vi "config_LS218_CRYO_FDS.vi"(8 "entrée d'erreur":errorcluster, 11 "Port_COM":refnum<visa-resource-name>) -> (0 "sortie d'erreur":errorcluster)   [LabVIEW 2016]
panel:
  out "conf_OK":bool
  out "conf_check":bool[](array[boolean])
  in  "VERIFIER CONFIG":bool
  out "LECTURE BUFFER":bool
  out "LOAD":string
  in  "Type sondes 5-8":u16(ring) items=["Diode 2.5V", "Diode 7.5V", "Pt < 250 Ohm", "Pt < 500 Ohm", "Pt < 5 KOhm", "Cernox"]
  in  "Type sondes 1-4":u16(ring) items=["Diode 2.5V", "Diode 7.5V", "Pt < 250 Ohm", "Pt < 500 Ohm", "Pt < 5 KOhm", "Cernox"]
  in  "Voies de mesures":T1(array[cluster]) {"Input_type" items=["aucune", "DT-470 (diode)", "DT-500 (diode)", "CTI (diode)", "DT- 670 (diode)", "Cernox", "Pt100", "Pt1000"]}
  out "nombre renvoyé":u32
  in  "SEND":bool
  out "RÉPONSE":string
  in  "COMMANDE":string
  in  "Celsius":bool
  in  "PÉRIODE ACQUISITION (sec)":i8(slide)=1 min=1 max=60 step=1 scale=1.0..60.0
  in  "NOM MANIP":string="Cryo FDS"
  in  "QUITTER":bool
  in  "DOSSIER":path=path "C:/Fete de la science"
  in  "Acquisition":bool
  # "ACQUISITION LAKESHORE 218 : CONFIGURATION"
  # "PARAMÈTRES D'ACQUISITION"
  # "J. HANSOTTE - IAS\nStation d'Étalonnage"
  # "ÉTAT LIAISON RS232"
  # "D'ENREGISTREMENT DES MESURES"
  # "UNITÉ"
  # "Kelvin"
  # "DEBUG"
  # "PARAMÈTRES DES VOIES DE MESURES"
  # "Nom des voies"
  # "Type de courbe"
  # "ON/OFF"
  # "T°"
  # "1"
  # "Liquéfacteur"
  # "2"
  # "3"
  # "4"
  # "Pompage LN2"
  # "5"
  # "6"
  # "7"
  # "8"
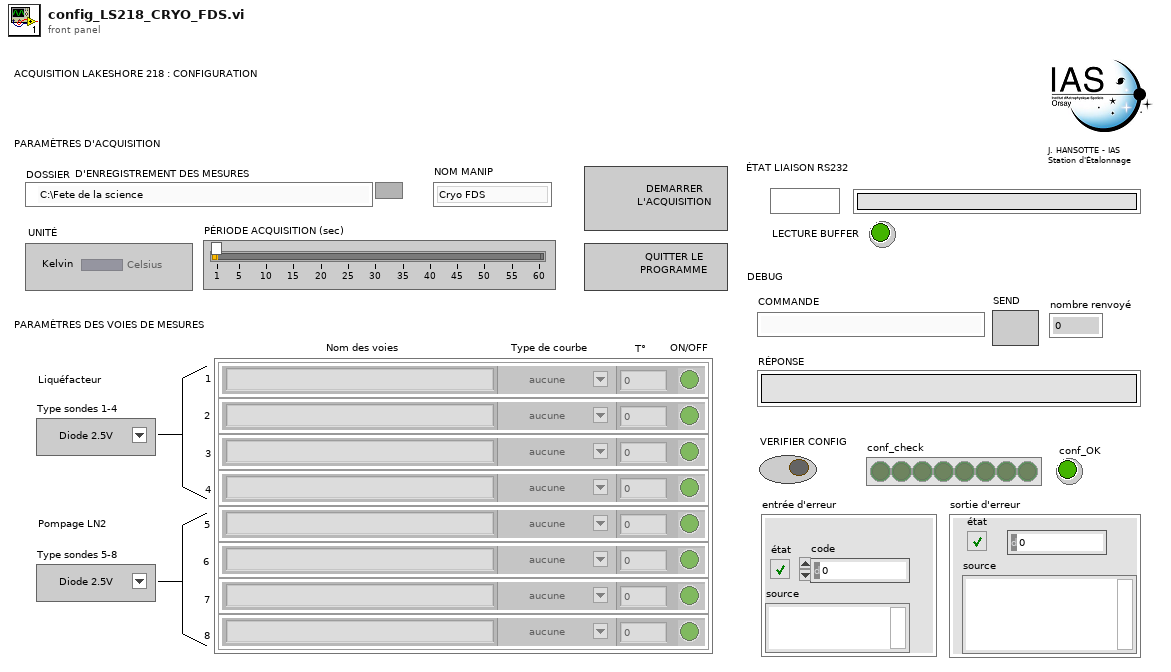
[diagram p1: front panel]
types:
  T1 = cluster{"Chaîne":string, "Input_type":u16, "Numérique":dbl, "Booléen":bool}[]
  T2 = cluster{"Chaîne":string, "CURVE_type":u16, "Numérique":dbl, "Booléen":bool}[]
  T3 = cluster{"Chaîne":string, "Input_type":u16, "Numérique":dbl, "Booléen":bool}
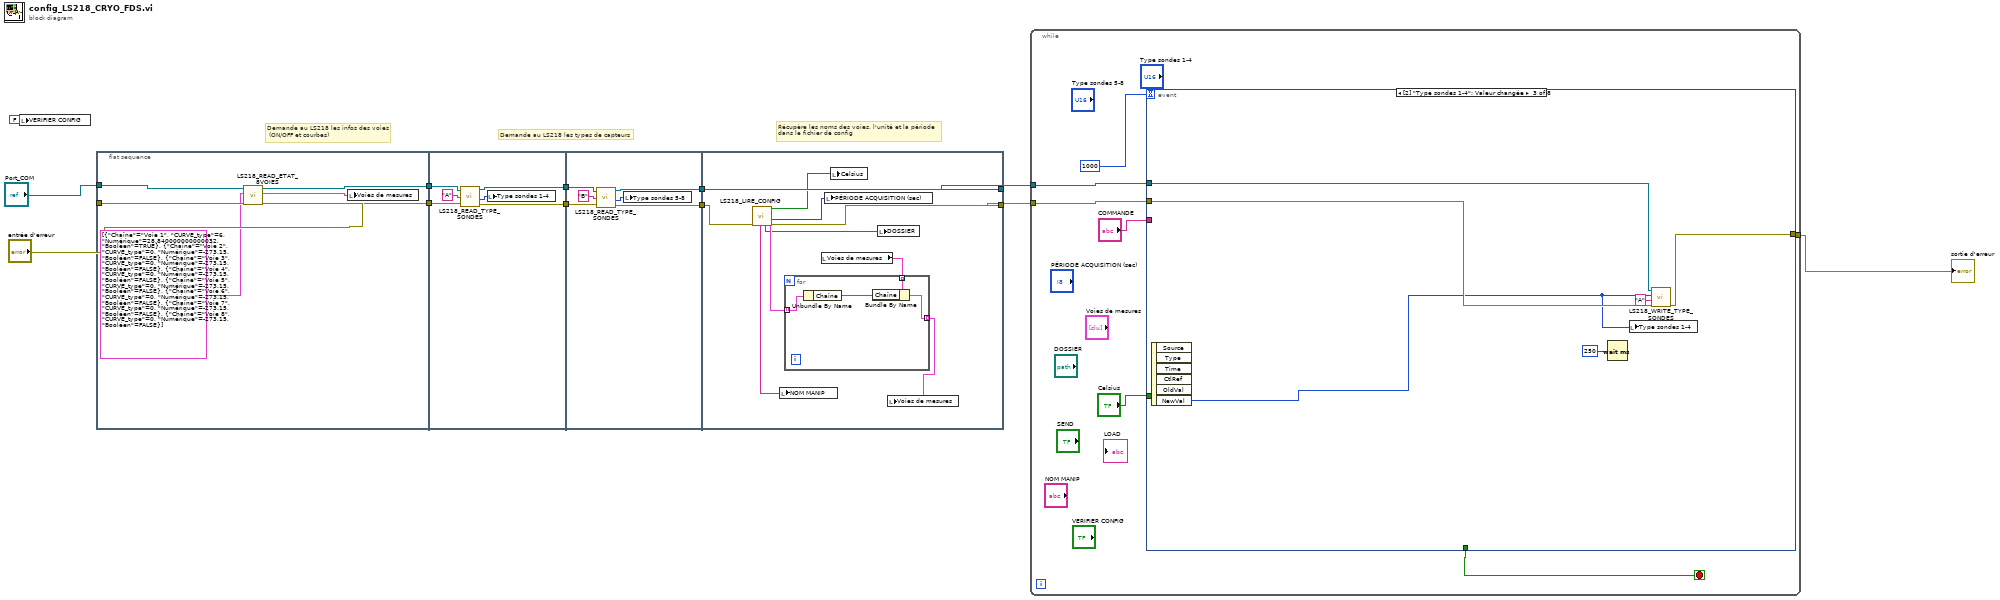
[diagram p0: block diagram]
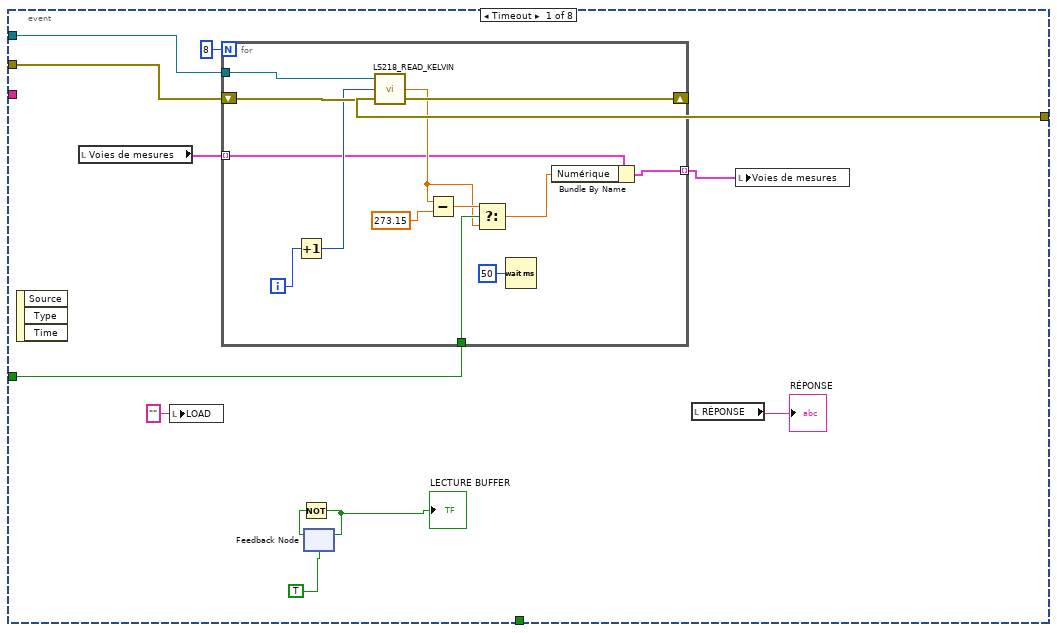
[diagram p2: hidden frame]
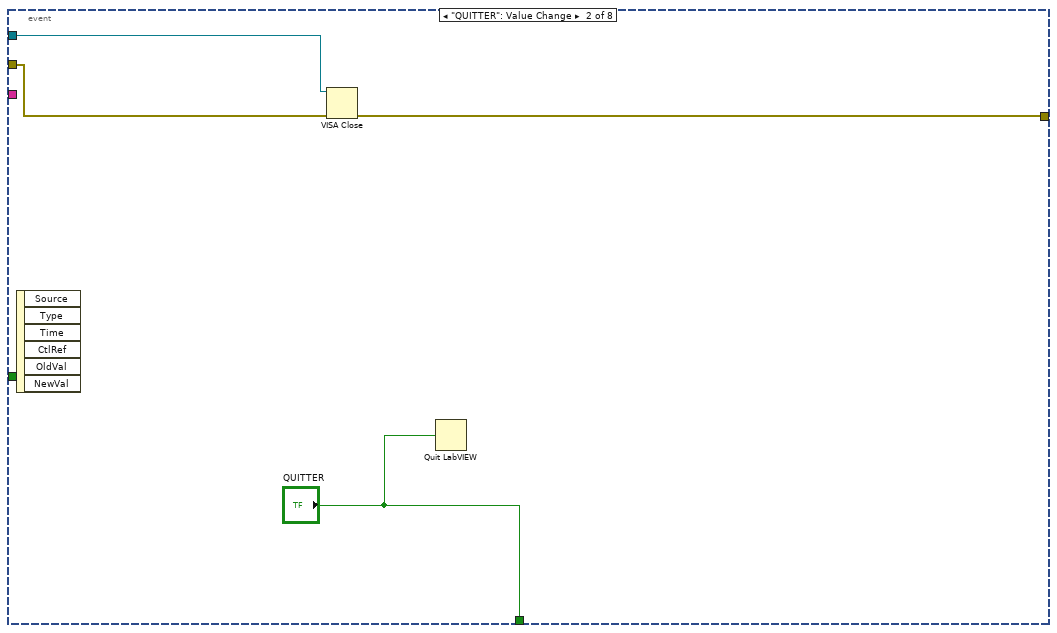
[diagram p3: hidden frame]
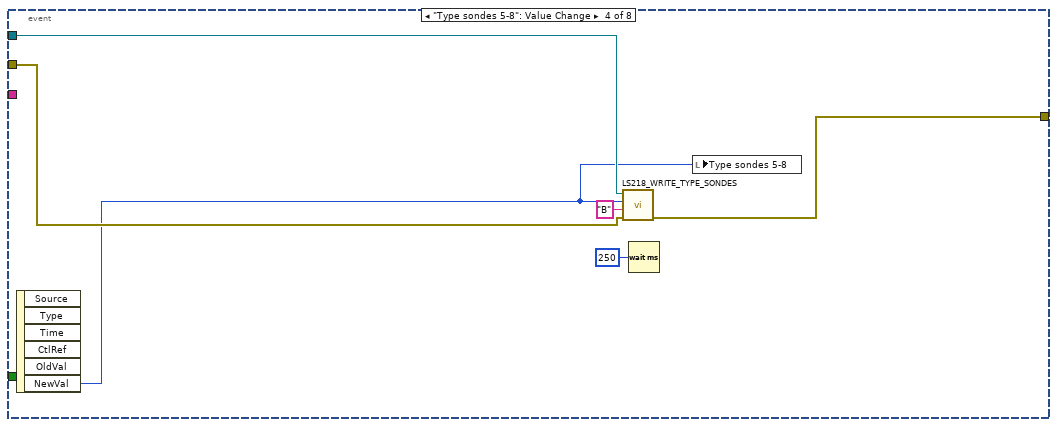
[diagram p4: hidden frame]
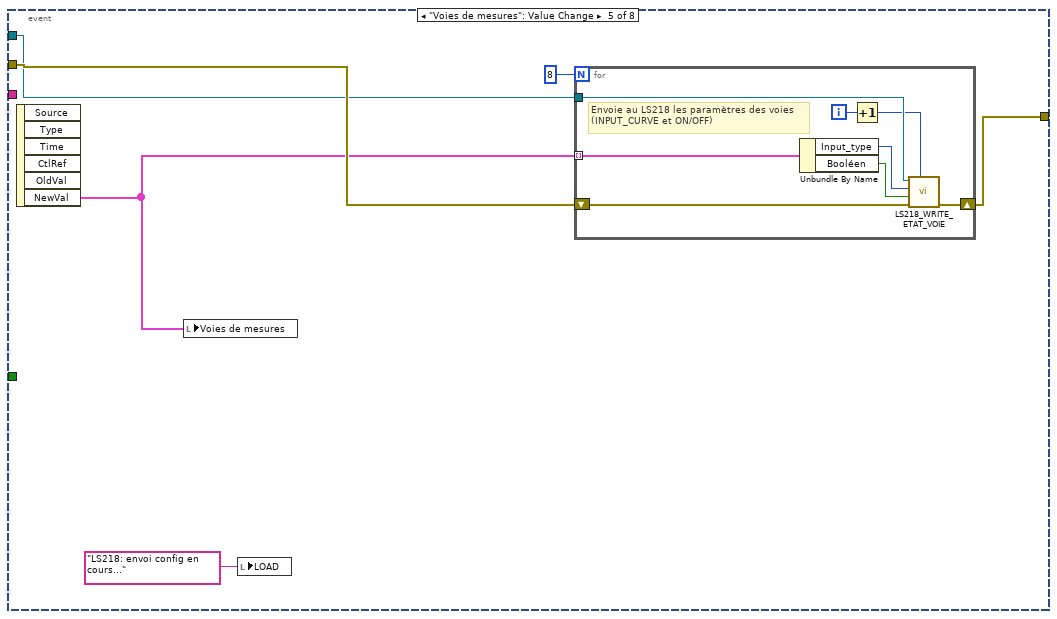
[diagram p5: hidden frame]
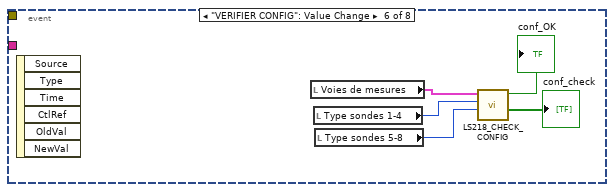
[diagram p6: hidden frame]
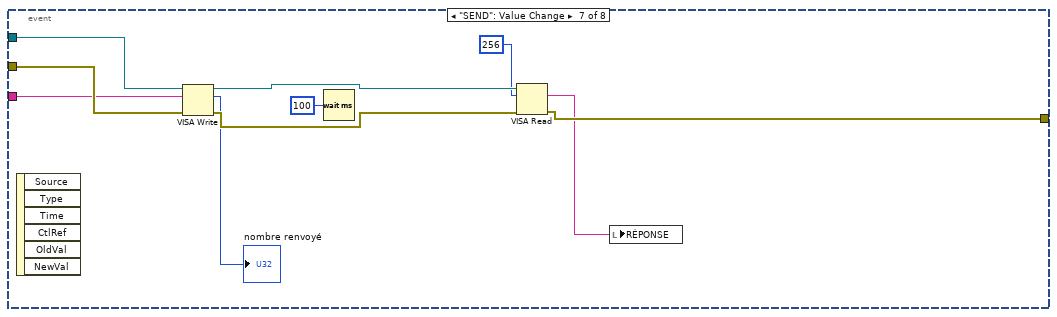
[diagram p7: hidden frame]
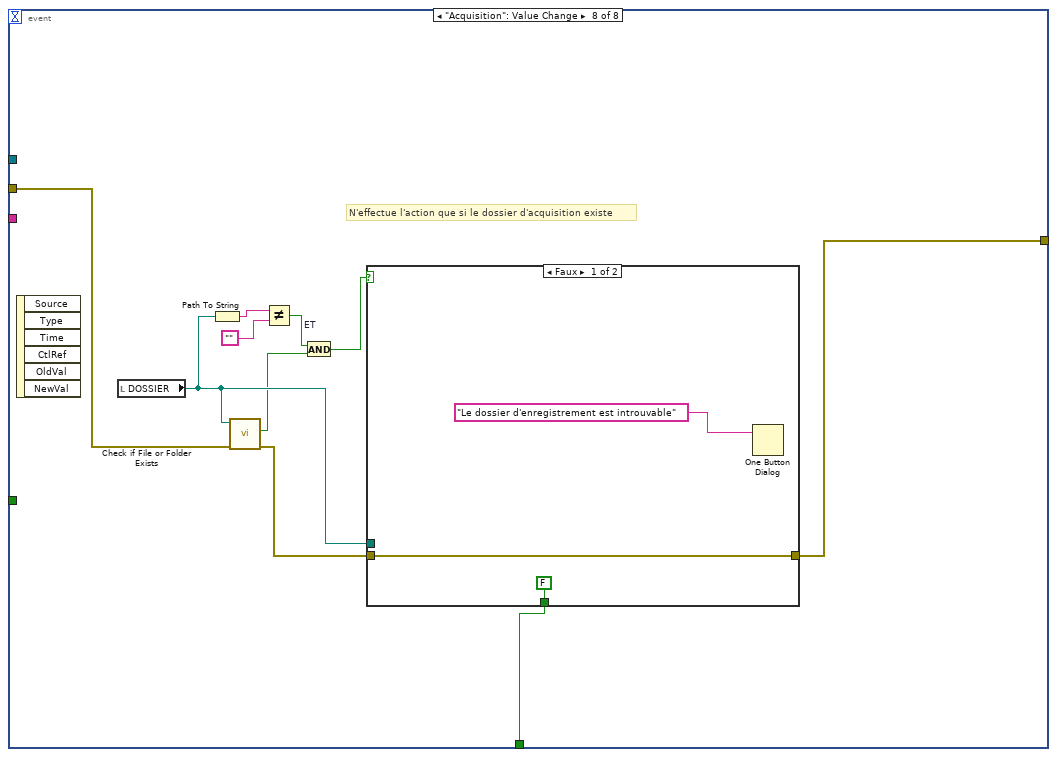
[diagram p8: hidden frame]
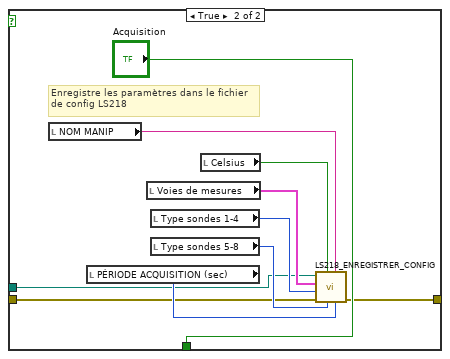
[diagram p9: hidden frame]
diagram:
  # "Récupère les noms des voies, l'unité et la période \ndans le fichier de config"
  # "Demande au LS218 les infos des voies\n (ON/OFF et courbes)"
  # "Demande au LS218 les types de capteurs"
  n1 = local write "VERIFIER CONFIG"(FALSE ("CONF CHECK")) -> ()
  n2 = flat-sequence {
    tunnel: [w17] -> w12
    tunnel: [w16] -> w11
    tunnel: "entrée d'erreur" -> [w18]
    tunnel: "Port_COM" -> [w14]
    tunnel: w12 -> [w23]
    tunnel: [w22] -> w10
    tunnel: w11 -> [w21]
    tunnel: [w20] -> w9
    tunnel: w10 -> [w29]
    tunnel: w9 -> [w27]
    tunnel: [w28] -> w4
    tunnel: [w26] -> w3
    tunnel: [w40] -> w7
    tunnel: [w37] -> w6
    tunnel: w4 -> [w38]
    tunnel: w3 -> [w40]
    frame #0 {
      n3 = call "LS218_READ_ETAT_8VOIES.vi"("entrée d'erreur"=w18, "Voies de mesures"=T2 [{"Chaîne"="Voie 1", "CURVE_type"=6, "Numérique"=28.840000000000032, "Booléen"=TRUE}, {"Chaîne"="Voie 2", "CURVE_type"=0, "Numérique"=-273.15, "Booléen"=FALSE}, {"Chaîne"="Voie 3", "CURVE_type"=0, "Numérique"=-273.15, "Booléen"=FALSE}, {"Chaîne"="Voie 4", "CURVE_type"=0, "Numérique"=-273.15, "Booléen"=FALSE}, {"Chaîne"="Voie 5", "CURVE_type"=0, "Numérique"=-273.15, "Booléen"=FALSE}, {"Chaîne"="Voie 6", "CURVE_type"=0, "Numérique"=-273.15, "Booléen"=FALSE}, {"Chaîne"="Voie 7", "CURVE_type"=0, "Numérique"=-273.15, "Booléen"=FALSE}, {"Chaîne"="Voie 8", "CURVE_type"=0, "Numérique"=-273.15, "Booléen"=FALSE}], "Refnum VISA en entrée"=w14) -> ("sortie d'erreur"=w17:errorcluster, "Tableau"=w15:T1, "Nom de ressource VISA en sortie"=w16:refnum<visa-resource-name>)  [unwired: 6 in]
      n4 = local write "Voies de mesures"(w15) -> ()
    }
    frame #1 {
      n5 = call "LS218_READ_TYPE_SONDES.vi"("Refnum VISA en entrée"=w21, "Voies A ou B"="A", "entrée d'erreur (pas d'erreur)"=w23) -> ("Nom de ressource VISA en sortie"=w20:refnum<visa-resource-name>, "Input_type"=w19:i32, "sortie d'erreur"=w22:errorcluster)  [unwired: 1 in]
      n6 = local write "Type sondes 1-4"(w19) -> ()
    }
    frame #2 {
      n7 = call "LS218_READ_TYPE_SONDES.vi"("Refnum VISA en entrée"=w27, "Voies A ou B"="B", "entrée d'erreur (pas d'erreur)"=w29) -> ("Nom de ressource VISA en sortie"=w26:refnum<visa-resource-name>, "Input_type"=w25:i32, "sortie d'erreur"=w28:errorcluster)  [unwired: 1 in]
      n8 = local write "Type sondes 5-8"(w25) -> ()
    }
    frame #3 {
      n9 = call "LS218_LIRE_CONFIG.vi"("entrée d'erreur (pas d'erreur)"=w38) -> ("sortie d'erreur"=w37:errorcluster, "PERIODE"=w32:i8, "Voies de mesures"=w39:T1, "Celsius"=w35:bool, "DOSSIER"=w36:path, "NOM MANIP"=w31:string)  [unwired: 3 in, 2 out]
      n10 = local write "NOM MANIP"(w31) -> ()
      n11 = local read "Voies de mesures"() -> (w33:T1)
      n12 = for {
        tunnel: w39 -> [w44] mode=indexing
        tunnel: [w42] -> w34 mode=indexing
        tunnel: w33 -> [w41] mode=indexing
        n13 = Unbundle By Name(w44) -> ("Chaîne"=w43:string)
        n14 = Bundle By Name(cluster=w41, "Chaîne"=w43) -> (w42:T3)
      }
      n15 = local write "PÉRIODE ACQUISITION (sec)"(w32) -> ()
      n16 = local write "Celsius"(w35) -> ()
      n17 = local write "DOSSIER"(w36) -> ()
      n18 = local write "Voies de mesures"(w34) -> ()
    }
  }
  n19 = while {
    tunnel: [w51] -> w2
    tunnel: w7 -> [w49]
    tunnel: w6 -> [w45]
    stop <- w50 stop-if-true
    n20 = event shown="[2] \"Type sondes 1-4\": Valeur changée" {
      selector: _ -> [_ _ _ _ _ _ _ _]
      dyn-events: _ -> [_ _ _ _ _ _ _ _]
      timeout: 1000 -> [_ _ _ _ _ _ _ _]
      tunnel: [w62 w77 w84 w90 w96 _ w118 w130] -> w51
      tunnel: [_ "QUITTER" _ _ _ _ _ w131] -> w50
      tunnel: w49 -> [w61 w79 w86 w92 w97 _ w117 _]
      tunnel: w45 -> [w60 w80 w85 w91 w98 _ w116 w129]
      tunnel: "COMMANDE" -> [_ _ _ _ _ _ w112 _]
      tunnel: "Celsius" -> [w59 _ _ _ _ _ _ _]
      event Timeout {
        n21 = event-data() -> ()  [unwired: 1 in, 3 out]
        n22 = local read "Voies de mesures"() -> (w56:T1)
        n23 = local write "LOAD"("" ("LOAD")) -> ()
        n24 = for {
          N: 8 -> [_]
          tunnel: w61 -> [w76]
          shift-right: [w67] -> w62
          shift-left: w60 -> [w75]
          tunnel: [w64] -> w58 mode=indexing
          tunnel: w59 -> [w73]
          tunnel: w56 -> [w66] mode=indexing
          i -> [w69]
          n25 = Increment(x=w69) -> (x+1=w68:i32)
          n26 = call "LS218_READ_KELVIN.vi"("entrée d'erreur (pas d'erreur)"=w75, "numéro voie"=w68, "Refnum VISA en entrée"=w76) -> ("sortie d'erreur"=w67:errorcluster, "T_Kelvin"=w71:dbl)  [unwired: 1 out]
          n27 = Subtract(x=w71, y=273.15) -> (x-y=w72:dbl)
          n28 = Select(t=w72, s=w73, f=w71) -> (s? t:f=w65:dbl)
          n29 = Wait (ms)(milliseconds to wait=u32 50 ("attente (ms)")) -> ()  [unwired: 1 out]
          n30 = Bundle By Name(cluster=w66, "Numérique"=w65) -> (w64:T3)
        }
        n31 = feedback #1(TRUE) -> (w53:bool)
        n32 = Not(x=w53) -> (.not. x?=w52:bool)
        "LECTURE BUFFER" <- w52
        n33 = feedback-in #1(w52) -> ()
        n34 = local read "RÉPONSE"() -> (→"RÉPONSE":string)
        n35 = local write "Voies de mesures"(w58) -> ()
      }
      event "QUITTER": Value Change {
        n36 = event-data() -> ()  [unwired: 1 in, 6 out]
        n37 = VISA Close(VISA resource name=w79, error in (no error)=w80) -> (error out=w77:errorcluster)
        n38 = Quit LabVIEW(quit? (T)="QUITTER") -> ()
      }
      event "Type sondes 1-4": Value Change {
        n39 = event-data() -> ("NewVal"=w83:u16)  [unwired: 1 in, 5 out]
        n40 = Wait (ms)(milliseconds to wait=u32 250 ("attente (ms)")) -> ()  [unwired: 1 out]
        n41 = local write "Type sondes 1-4"(w83) -> ()
        n42 = call "LS218_WRITE_TYPE_SONDES.vi"("entrée d'erreur (pas d'erreur)"=w85, "A ou B"="A", "Input_type"=w83, "Refnum VISA en entrée"=w86) -> ("sortie d'erreur"=w84:errorcluster)  [unwired: 2 in, 1 out]
      }
      event "Type sondes 5-8": Value Change {
        n43 = event-data() -> ("NewVal"=w89:u16)  [unwired: 1 in, 5 out]
        n44 = call "LS218_WRITE_TYPE_SONDES.vi"("entrée d'erreur (pas d'erreur)"=w91, "A ou B"="B", "Input_type"=w89, "Refnum VISA en entrée"=w92) -> ("sortie d'erreur"=w90:errorcluster)  [unwired: 2 in, 1 out]
        n45 = Wait (ms)(milliseconds to wait=u32 250 ("attente (ms)")) -> ()  [unwired: 1 out]
        n46 = local write "Type sondes 5-8"(w89) -> ()
      }
      event "Voies de mesures": Value Change {
        n47 = event-data() -> ("NewVal"=w94:T1)  [unwired: 1 in, 5 out]
        n48 = local write "Voies de mesures"(w94) -> ()
        n49 = local write "LOAD"("LS218: envoi config en cours..." ("LOAD")) -> ()
        n50 = for {
          N: 8 -> [_]
          shift-right: [w104] -> w96
          shift-left: w98 -> [w105]
          tunnel: w97 -> [w103]
          tunnel: w94 -> [w100] mode=indexing
          i -> [w106]
          # "Envoie au LS218 les paramètres des voies \n(INPUT_CURVE et ON/OFF)"
          n51 = Unbundle By Name(w100) -> ("Input_type"=w99:u16, "Booléen"=w101:bool)
          n52 = Increment(x=w106) -> (x+1=w102:i32)
          n53 = call "LS218_WRITE_ETAT_VOIE.vi"("numéro voie"=w102, "entrée d'erreur (pas d'erreur)"=w105, "INPUT ON"=w101, "Input_curve"=w99, "Refnum VISA en entrée"=w103) -> ("sortie d'erreur"=w104:errorcluster)  [unwired: 2 in, 1 out]
        }
      }
      event "VERIFIER CONFIG": Value Change {
        n54 = event-data() -> ()  [unwired: 1 in, 6 out]
        n55 = local read "Voies de mesures"() -> (w111:T1)
        n56 = local read "Type sondes 1-4"() -> (w110:u16)
        n57 = local read "Type sondes 5-8"() -> (w109:u16)
        n58 = call "LS218_CHECK_CONFIG.vi"("Type sondes 5-8"=w109, "Type sondes 1-4"=w110, "table_voies"=w111) -> ("conf_check"=→"conf_check":bool[], "conf_OK"=→"conf_OK":bool)  [unwired: 4 in, 2 out]
      }
      event "SEND": Value Change {
        n59 = event-data() -> ()  [unwired: 1 in, 6 out]
        n60 = VISA Write(VISA resource name=w117, write buffer=w112, error in (no error)=w116) -> (VISA resource name out=w121:refnum<visa-resource-name>, return count=→"nombre renvoyé":u32, error out=w119:errorcluster)
        n61 = Wait (ms)(milliseconds to wait=u32 100 ("attente (ms)")) -> ()  [unwired: 1 out]
        n62 = VISA Read(VISA resource name=w121, byte count=u32 256 ("nombre d'octets"), error in (no error)=w119) -> (read buffer=w113:string, error out=w118:errorcluster)  [unwired: 2 out]
        n63 = local write "RÉPONSE"(w113) -> ()
      }
      event "Acquisition": Value Change {
        # "N'effectue l'action que si le dossier d'acquisition existe"
        n64 = event-data() -> ()  [unwired: 1 in, 6 out]
        n65 = local read "DOSSIER"() -> (w127:path)
        n66 = Path To String(path=w127) -> (string=w126:string)
        n67 = call <vilib>:"Check if File or Folder Exists.vi"("error in (no error)"=w129, "path"=w127) -> ("error out"=w128:errorcluster, "file or folder exists?"=w124:bool)  [unwired: 7 in, 1 out]
        n68 = Not Equal?(x=w126, y="") -> (x != y?=w123:bool)
        n69 = And "ET"(x=w123, y=w124) -> (x .and. y?=w122:bool)
        n70 = case shown="Faux" w122 {
          tunnel: [FALSE ("Acquisition") "Acquisition"] -> w131
          tunnel: [w134 w137] -> w130
          tunnel: w127 -> [_ w136]
          tunnel: w128 -> [w134 w135]
          frame False {
            n71 = One Button Dialog(message="Le dossier d'enregistrement est introuvable") -> ()  [unwired: 1 in, 1 out]
          }
          frame True {
            # "Enregistre les paramètres dans le fichier\nde config LS218"
            n72 = local read "NOM MANIP"() -> (w138:string)
            n73 = local read "PÉRIODE ACQUISITION (sec)"() -> (w139:i8)
            n74 = local read "Voies de mesures"() -> (w141:T1)
            n75 = local read "Type sondes 1-4"() -> (w142:u16)
            n76 = local read "Type sondes 5-8"() -> (w143:u16)
            n77 = local read "Celsius"() -> (w140:bool)
            n78 = call "LS218_ENREGISTRER_CONFIG.vi"("periode_acqui"=w139, "NOM MANIP"=w138, "Type sondes 5-8"=w143, "Celsius"=w140, "entrée d'erreur (pas d'erreur)"=w135, "Type sondes 1-4"=w142, "Voies de mesures"=w141, "DOSSIER"=w136) -> ("sortie d'erreur"=w137:errorcluster)  [unwired: 3 in]
          }
        }
      }
    }
  }
  "sortie d'erreur" <- w2
